vi "build event cluster BAE2.vi"(1 "time cluster in":T1, 2 "position in [km]":sgl) -> (8 "event data out":T2)   [LabVIEW 2014]
doc: "Build Event Cluster\n\nTakes position [km] and time [nsec] and bundles it into an evnt cluster.\n\nBeverly Abadines\nPHY 350\nE2"
uses:
  typedefs/event cluster typedef.ctl
  typedefs/time cluster typedef.ctl
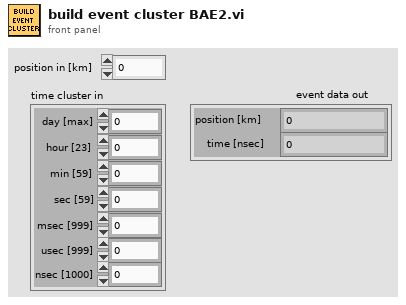
[diagram p1: front panel]
types:
  T1 = typedef "time cluster typedef.ctl" = cluster{"day [max]":u32, "hour [23]":u32, "min [59]":u32, "sec [59]":u32, "msec [999]":u32, "usec [999]":u32, "nsec [1000]":u32}
  T2 = typedef "event cluster typedef.ctl" = cluster{"position [km]":sgl, "time [nsec]":i64}
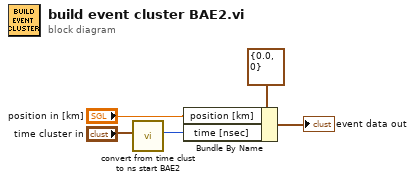
[diagram p0: block diagram]
diagram:
  n1 = call "convert from time clust to ns start BAE2.vi"("time cluster"="time cluster in") -> ("time (nsec)"=w1:i64)  [unwired: 9 in]
  n2 = Bundle By Name(cluster=T2 {"position [km]"=0.0, "time [nsec]"=0} ("event data out"), "position [km]"="position in [km]", "time [nsec]"=w1) -> (→"event data out":T2)
